vi "Add LabVIEW Error.vi"(8 "error in (no error)":errorcluster) -> (0 "error out":errorcluster)   [LabVIEW 2021, in "Error Handler Actor API.lvclass"]
uses:
  Error Handler Actor API.lvclass
  Re-use Libraries/Minimal Actor Framework/Messaging/Message/Message.lvclass
  Error Handler Actor API.lvclass/Error Handler Actor API.ctl
  Globals.vi
  Re-use Libraries/Utility/Utility.lvlib
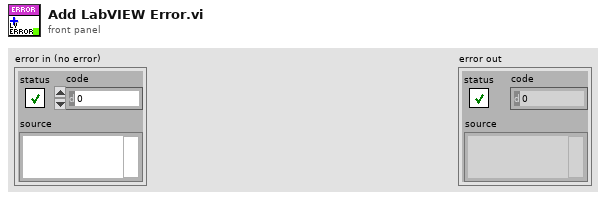
[diagram p1: front panel]
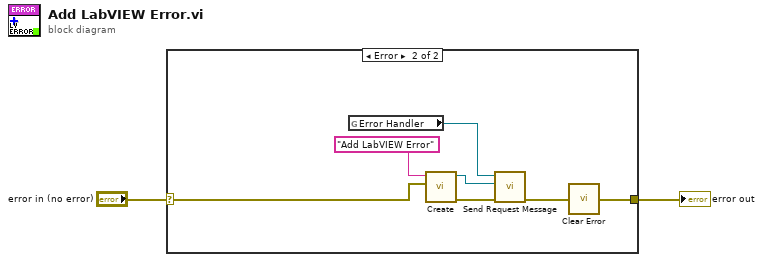
[diagram p0: block diagram]
diagram:
  n1 = case shown="Error" "error in (no error)" {
    selector: "error in (no error)" -> [w3 w4]
    tunnel: [w3 w5] -> w2
    frame No Error {
    }
    frame Error {
      n2 = global read "Globals.vi" "Error Handler"() -> (w6:refnum<class "Error Handler Actor API.lvclass">)
      n3 = call "Create.vi"("Data"=w4, "Name"="Add LabVIEW Error" ("Parameter")) -> ("error out"=w7:errorcluster, "Message out"=w8:refnum<class "Message.lvclass">)  [unwired: 8 in]
      n4 = call-dynamic "Send Request Message.vi"("error in (no error)"=w7, "Message"=w8, "Actor API in"=w6) -> ("error out"=w10:errorcluster)  [unwired: 8 in]
      n5 = call "Clear Error.vi"("error in (no error)"=w10) -> ("error out"=w5:errorcluster)
    }
  }
  "error out" <- w2
